vi "Preset.vi"(8 "error in (no error)":errorcluster {"code" format="%.0x"}, 9 "RadioStandard (B1M4)":i32(ring) items=["B1M4", "B3M", "B5M", "B10M", "B15M", "B20M", "Preset Standarddtv16", "Preset Standarddvb16", "Preset Standarddvb32", "Preset Standarddvb64", "Preset Standardap 1c 4fm", "Preset Standardap 1cqpsk", "Preset Standardap 2hcpm", "Preset Standardap 2hdqpsk", "Preset Standardap 2hdqpskevm", "Preset Standarddmr", "Preset Standarddpmr", "Preset Standarddect", "Preset Standardtetra", "Preset Standardvdl2", "Preset Standardmilstdcpm", "Preset Standardws 2f5 0k1", "Preset Standardws 2f10 0k1", "Preset Standardws 2f10 0k05", "Preset Standardws 2f15 0k05", "Preset Standardws 2f20 0k1", "Preset Standardws 2f20 0k05", "Preset Standardws 2f30 0k05", "Preset Standardsoqpsktg"], 11 "instrument handle":refnum<k15>) -> (0 "error out":errorcluster {"code" format="%.0x"}, 3 "instrument handle out":refnum<k15>)   [LabVIEW 2021, in "Keysight XSAnVMA.lvlib"]
doc: "Sets the parameters to the LTE standard."
uses:
  <instrlib>/Keysight XSAnVMA/Keysight XSAnVMA.lvlib
  KtXSAnVMA_64.dll
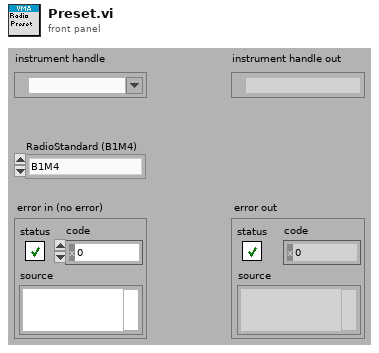
[diagram p1: front panel]
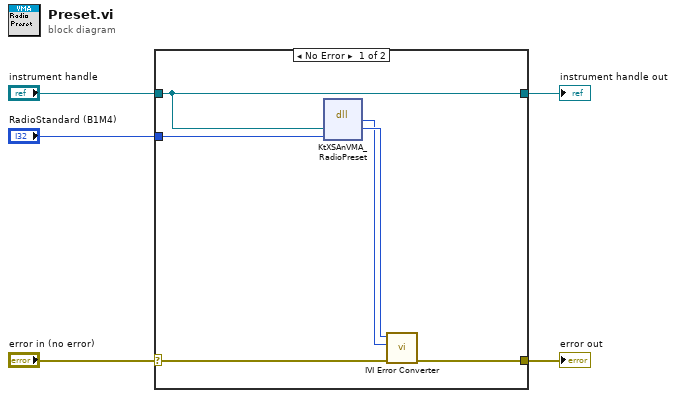
[diagram p0: block diagram]
diagram:
  n1 = case shown="No Error" "error in (no error)" {
    selector: "error in (no error)" -> [w9 w13]
    tunnel: [w8 w13] -> w5
    tunnel: "instrument handle" -> [w6 w12]
    tunnel: "RadioStandard (B1M4)" -> [w7 _]
    tunnel: [w6 w12] -> w1
    frame No Error {
      n2 = dll-call lib="KtXSAnVMA**.dll" fn="KtXSAnVMA_RadioPreset"("Vi"=w6, "RadioStandard"=w7) -> (w10:i32, "Vi"=w11:u32)  [unwired: 4 in, 2 out]
      n3 = call <instrlib>:"IVI Error Converter.vi"("error in (no error)"=w9, "IVI error code (0)"=w10, "instrument handle"=w11) -> ("error out"=w8:errorcluster)  [unwired: 7 in, 1 out]
    }
    frame Error {
    }
  }
  "error out" <- w5
  "instrument handle out" <- w1
